vi "chart title set overlay.vi"(8 "error in (no error)":errorcluster, 10 "overlay":u8, 11 "chart":u32) -> (0 "error out":errorcluster)   [LabVIEW 8.6]
doc: "void chart_title_set_overlay(lxw_chart chart, uint8_t overlay);"
uses:
  pending_lvxlsxwriter/xlsxwriter.dll
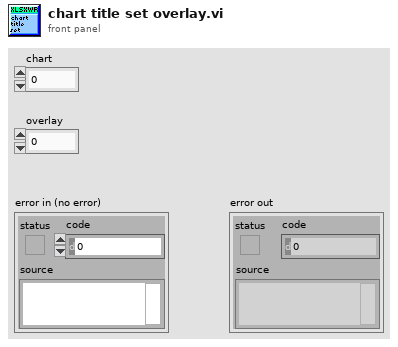
[diagram p1: front panel]
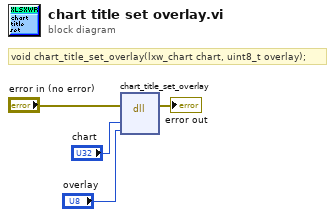
[diagram p0: block diagram]
diagram:
  # "void chart_title_set_overlay(lxw_chart chart, uint8_t overlay);"
  n1 = dll-call lib="C:/Users/WDAGUtilityAccount/Desktop/pending_lvxlsxwriter/xlsxwriter.*" fn="chart_title_set_overlay"(error in="error in (no error)", "chart"="chart", "overlay"="overlay") -> (error out=→"error out":errorcluster)  [unwired: 5 in, 1 out]
